vi "TT Settings Dialog.vi"(8 "error in (no error)":errorcluster, 11 "TT Module Config in":T2) -> (0 "error out":errorcluster, 1 "Cancelled?":bool=TRUE, 2 "UI Refresh Needed?":bool, 3 "TT Module Config out":T2)   [LabVIEW 2018, in "TT Module.lvlib"]
doc: "Dialog for selecting user specified settings."
uses:
  TT Module.lvlib
  Controls/TT Module Config Cluster.ctl
  <vilib>/Utility/miscctls.llb/LVPoint32TypeDef.ctl
  Tag VIs/Numeric Alarm Settings Cluster.ctl
  PT Module/Controls/PT Settings Dialog.ctl
  Tag VIs/Tag FGV Operation Enum.ctl
  Shared Variables/Simple Alarm Values Cluster.ctl
  Shared Variables/Dynamic Shared Variables.lvlib
  PT Module/PT Module.lvlib
panel:
  in  "Module Name":string
  in  "Settings Dialog":T1 {"Input Channel Tag Name" items=["Temperature", "Temperature_0"]}
  in  "Cancel Button":bool
  in  "OK Button":bool
  # "Non visible portion of dialog (needed for connector pane)."
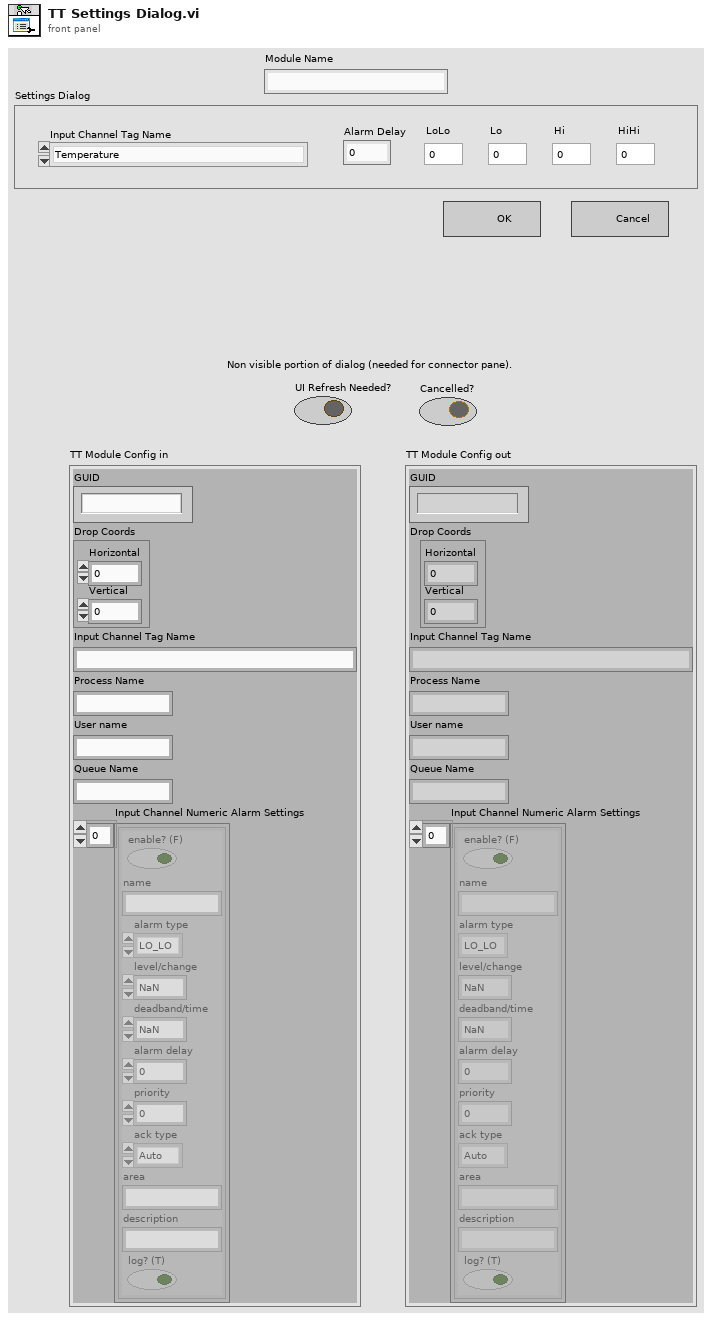
[diagram p1: front panel]
types:
  T1 = typedef "PT Module.lvlib/PT Settings Dialog.ctl" = cluster{"Input Channel Tag Name":u16, "LoLo":dbl, "Lo":dbl, "Hi":dbl, "HiHi":dbl, "Alarm Delay":dbl}
  T2 = typedef "TT Module.lvlib/TT Module Config Cluster.ctl" = cluster{"GUID":string, "Drop Coords":T3, "Input Channel Tag Name ":string, "Process Name":string, "User name":string, "Queue Name":string, "Input Channel Numeric Alarm Settings":T4[]}
  T3 = typedef "LVPoint32TypeDef.ctl" = cluster{"Horizontal":i32, "Vertical":i32}
  T4 = typedef "Numeric Alarm Settings Cluster.ctl" = cluster{"enable? (F)":bool, "name":string, "alarm type":enum16{"HI_HI", "HI", "LO", "LO_LO"}, "level/change":dbl, "deadband/time":dbl, "alarm delay":dbl, "priority":u32, "ack type":enum16{"Auto", "User", "None", "Each Occurrence"}, "area":string, "description":string, "log? (T)":bool}
  T5 = typedef "Tag FGV Operation Enum.ctl" = enum16{"Init", "Set Notification Queue", "Create Tag", "Commit", "Write Tag (Numeric)", "Write Tag (Boolean)", "Read All Tags", "Read One Tag", "Delete Tag Category", "Set Alarm Parameters (Numeric)", "Set Alarm Parameters (Boolean)", "Enable All Alarms", "Disable All Alarms", "Delete All Tags", "Read Alarms", "Ack Alarm", "Read Alarm Parameters (Numeric)", "Read Alarm Parameters (Boolean)"}
  T6 = typedef "Dynamic Shared Variables.lvlib/Simple Alarm Values Cluster.ctl" = cluster{"tag name":string, "HiHi":dbl, "Hi":dbl, "Lo":dbl, "LoLo":dbl, "alarm delay":dbl}
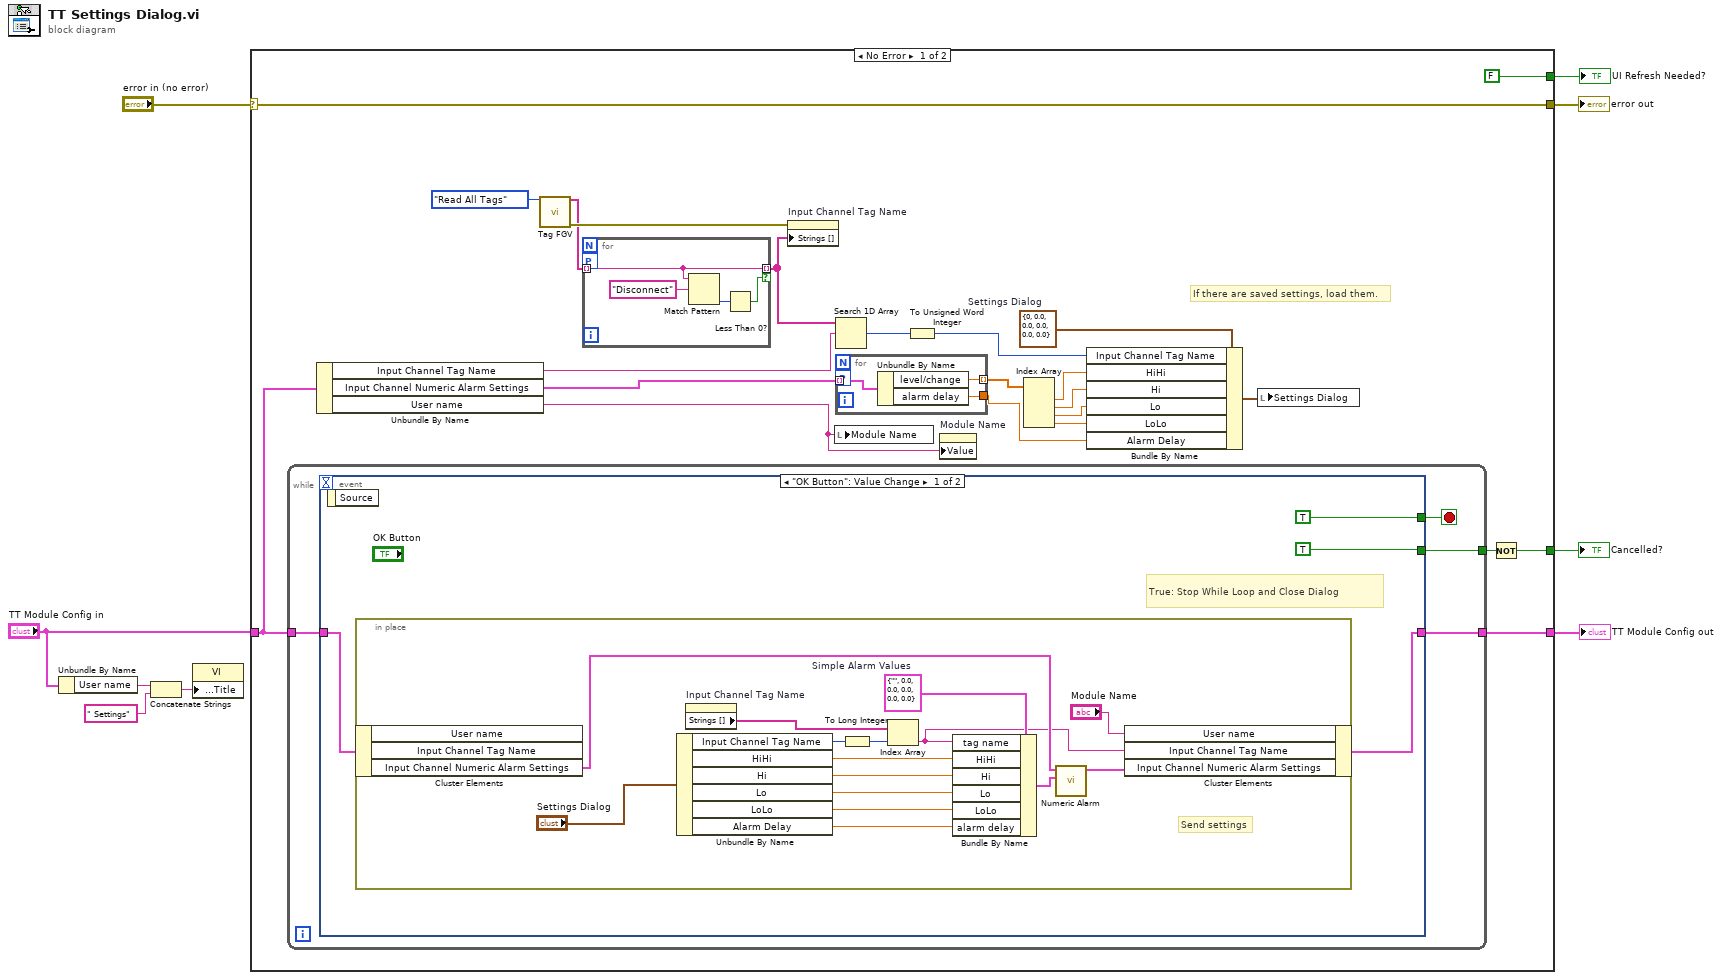
[diagram p0: block diagram]
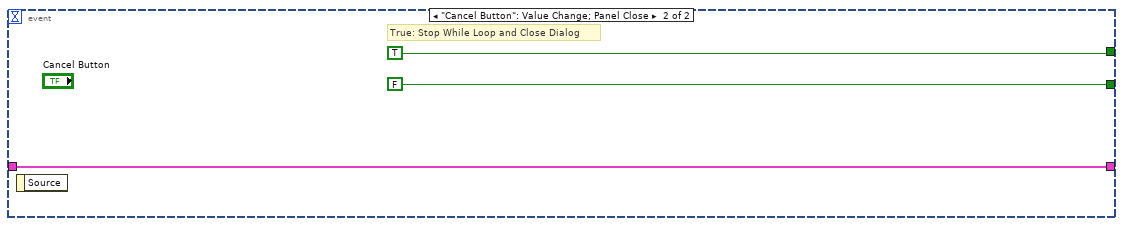
[diagram p2: hidden frame]
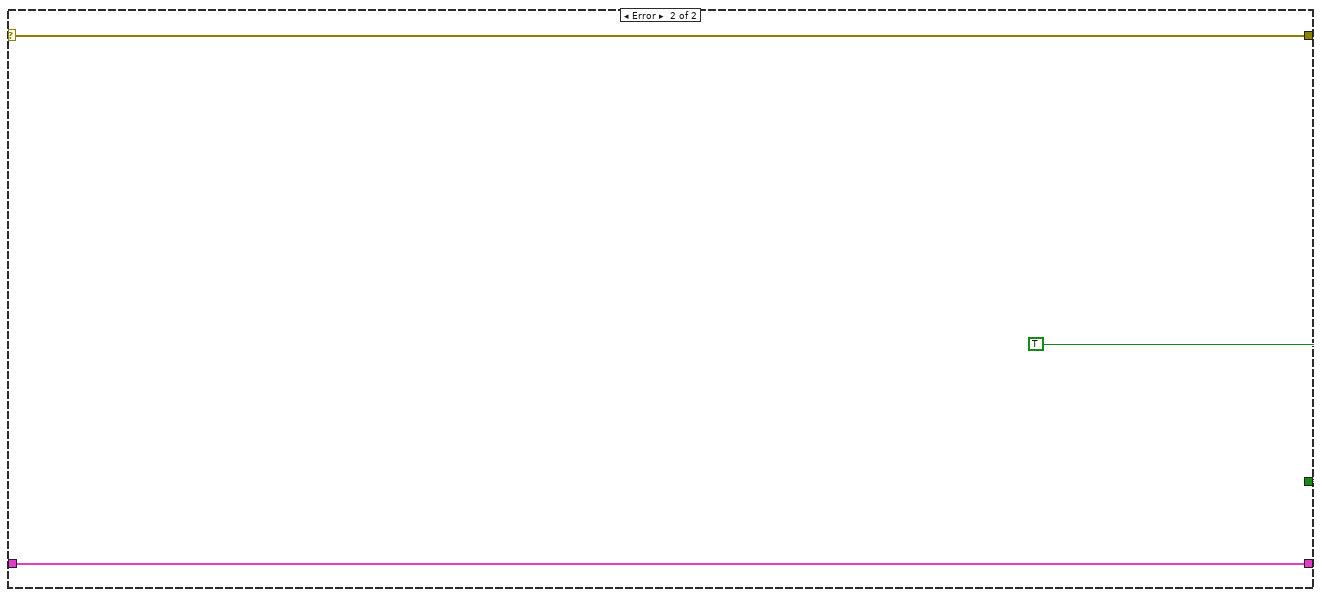
[diagram p3: hidden frame]
diagram:
  n1 = Unbundle By Name("TT Module Config in") -> ("User name"=w2:string)
  n2 = Concatenate Strings(w2, " Settings" ("string")) -> (w4:string)
  n3 = property class="VI"("Front Panel.Title"=w4) -> ()  [unwired: 2 in, 2 out]
  n4 = case shown="No Error" "error in (no error)" {
    selector: "error in (no error)" -> [w32 w68]
    tunnel: [w32 w68] -> w9
    tunnel: "TT Module Config in" -> [w29 w67]
    tunnel: [w30 w67] -> w5
    tunnel: [FALSE ("UI Refresh Needed?") _] -> w8
    tunnel: [w27 TRUE ("UI Refresh Needed?")] -> w7
    frame No Error {
      w23 = T1 {"Input Channel Tag Name"=0, "LoLo"=0.0, "Lo"=0.0, "Hi"=0.0, "HiHi"=0.0, "Alarm Delay"=0.0}  # Settings Dialog
      # "If there are saved settings, load them."
      n5 = while {
        tunnel: [w43] -> w28
        tunnel: [w40] -> w30
        tunnel: w29 -> [w42]
        stop <- w41 stop-if-true
        n6 = event shown="[0] \"OK Button\": Value Change" {
          selector: _ -> [_ _]
          dyn-events: _ -> [_ _]
          timeout: _ -> [_ _]
          tunnel: w42 -> [w45 w65]
          tunnel: [TRUE ("UI Refresh Needed?") FALSE ("UI Refresh Needed?")] -> w43
          tunnel: [TRUE TRUE] -> w41
          tunnel: [w44 w65] -> w40
          event "OK Button": Value Change {
            # "True: Stop While Loop and Close Dialog"
            n7 = event-data() -> ()  [unwired: 1 in, 1 out]
            n8 = in-place {
              w54 = T6 {"tag name"="", "HiHi"=0.0, "Hi"=0.0, "Lo"=0.0, "LoLo"=0.0, "alarm delay"=0.0}  # Simple Alarm Values
              # "Send settings"
              n9 = in-place-cluster #1(w45) -> ("Input Channel Numeric Alarm Settings"=w51:T4[])  [unwired: 2 out]
              n10 = Unbundle By Name("Settings Dialog") -> ("Input Channel Tag Name"=w60:u16, "HiHi"=w58:dbl, "Hi"=w57:dbl, "Lo"=w56:dbl, "LoLo"=w55:dbl, "Alarm Delay"=w52:dbl)
              n11 = property on="Input Channel Tag Name" class="Ring (strict)"() -> ("Strings []"=w61:string[])  [unwired: 2 in, 2 out]
              n12 = To Long Integer(number=w60) -> (32bit integer=w59:i32)
              n13 = Index Array(array=w61, index=w59) -> (element=w49:string)
              n14 = Bundle By Name(cluster=w54, "tag name"=w49, "HiHi"=w58, "Hi"=w57, "Lo"=w56, "LoLo"=w55, "alarm delay"=w52) -> (w53:T6)
              n15 = call "Numeric Alarm.vi"("Simple Alarm Values"=w53, "Alarms in"=w51) -> ("Alarms out"=w48:T4[])  [unwired: 9 in]
              n16 = in-place-cluster #1("User name"="Module Name", "Input Channel Tag Name"=w49, "Input Channel Numeric Alarm Settings"=w48) -> (w44:T2)
            }
          }
          event "Cancel Button": Value Change; Panel Close {
            # "True: Stop While Loop and Close Dialog"
            n17 = event-data() -> ()  [unwired: 1 in, 1 out]
          }
        }
      }
      n18 = Unbundle By Name(w29) -> ("Input Channel Tag Name"=w26:string, "Input Channel Numeric Alarm Settings"=w24:T4[], "User name"=w15:string)
      n19 = call "Tag FGV.vi"("Operation"=Tag_FGV_Operation_Enum."Read All Tags") -> ("Tag Names"=w12:string[], "error out"=w13:errorcluster)  [unwired: 7 in, 6 out]
      n20 = for {
        tunnel: w12 -> [w34] mode=indexing
        tunnel: [w34] -> w11 mode=indexing if=w33
        workers-P: _ -> [_]
        n21 = Match Pattern(string=w34, regular expression="Disconnect" ("name")) -> (offset past match=w36:i32)  [unwired: 1 in, 3 out]
        n22 = Less Than 0?(x=w36) -> (x < 0?=w33:bool)
      }
      n23 = property on="Input Channel Tag Name" class="Ring (strict)"(error in=w13, "Strings []"=w11) -> ()  [unwired: 1 in, 2 out]
      n24 = local write "Module Name"(w15) -> ()
      n25 = Search 1D Array(1D array=w11, element=w26) -> (index of element=w25:i32)  [unwired: 1 in]
      n26 = for {
        tunnel: w24 -> [w39] mode=indexing
        tunnel: [w38] -> w20 mode=indexing
        tunnel: [w37] -> w10
        workers-P: _ -> [_]
        n27 = Unbundle By Name(w39) -> ("level/change"=w38:dbl, "alarm delay"=w37:dbl)
      }
      n28 = To Unsigned Word Integer(number=w25) -> (unsigned 16bit integer=w22:u16)
      n29 = property on="Module Name" class="Str"("Value"=w15) -> ()  [unwired: 2 in, 2 out]
      n30 = Index Array(array=w20) -> (element #1=w19:dbl, element #2=w18:dbl, element #3=w17:dbl, element #4=w16:dbl)  [unwired: 4 in]
      n31 = Bundle By Name(cluster=w23, "Input Channel Tag Name"=w22, "HiHi"=w19, "Hi"=w18, "Lo"=w17, "LoLo"=w16, "Alarm Delay"=w10) -> (w21:T1)
      n32 = local write "Settings Dialog"(w21) -> ()
      n33 = Not(x=w28) -> (.not. x?=w27:bool)
    }
    frame Error {
    }
  }
  "UI Refresh Needed?" <- w8
  "error out" <- w9
  "TT Module Config out" <- w5
  "Cancelled?" <- w7
